vi "Simple TCP - Server - Copy 3 - Copy.vi"() -> ()   [LabVIEW 2021]
doc: "Demonstrates how to set up a basic TCP connection, send data to the specified port once a connection has been established, and terminate the connection once the data has been sent. This VI is designed to stop if the TCP connection is terminated. The data sent in this example is an array of random numbers."
uses:
  <vilib>/Analysis/3filter.llb/Filter Passband Type.ctl
  <vilib>/Analysis/5stat.llb/RMS (DBL).vi
  <vilib>/Analysis/3filter.llb/Butterworth Filter (DBL).vi
  <vilib>/Analysis/NI_AALBase.lvlib
  <vilib>/Analysis/NI_AALPro.lvlib
panel:
  out "Numeric":dbl
  in  "Client Closed":string="The client VI closed the connection."
  out "Waveform Graph":dbl[](graph)
  in  "Stop":bool
  # "Overview: Demonstrates the use of the TCP functions to initialize a TCP server that can send data to a client VI.\nInstructions:\n1. Run the VI.\n2. Open Simple TCP - Client.vi and follow the instructions on its front panel. Note that if you wait longer than 30 seconds to do this after running this VI, it will time out.\n3. Click Stop to stop the VI. Note that if you stop the client VI, this VI will stop automatically."
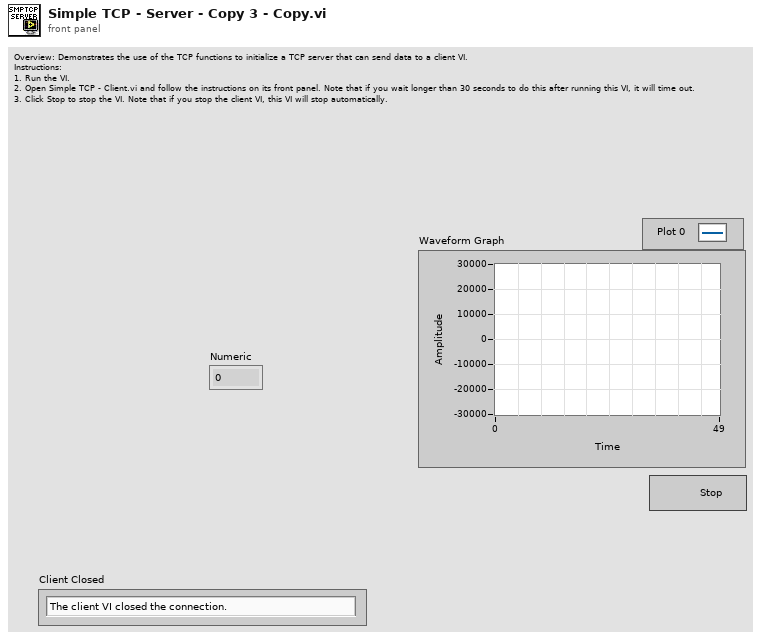
[diagram p1: front panel]
types:
  T1 = typedef "NI_AALBase.lvlib/Filter Passband Type.ctl" = enum32{"Lowpass", "Highpass", "Bandpass", "Bandstop"}
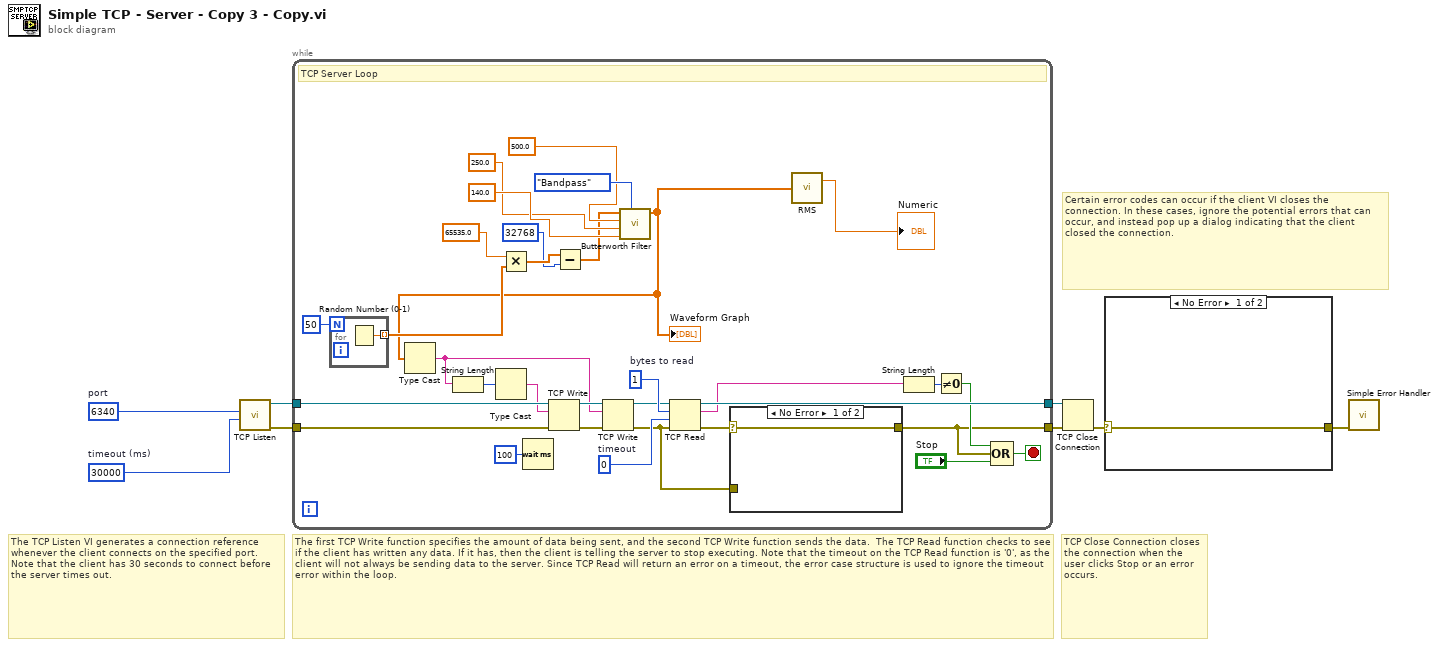
[diagram p0: block diagram]
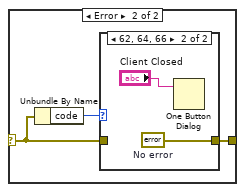
[diagram p2: hidden frame]
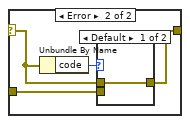
[diagram p4: hidden frame]
diagram:
  w1 = u16 6340  # port
  w2 = 30000  # timeout (ms)
  # "TCP Close Connection closes the connection when the user clicks Stop or an error occurs."
  # "The TCP Listen VI generates a connection reference whenever the client connects on the specified port. Note that the client has 30 seconds to connect before the server times out."
  # "Certain error codes can occur if the client VI closes the connection. In these cases, ignore the potential errors that can occur, and instead pop up a dialog indicating that the client closed the connection."
  # "The first TCP Write function specifies the amount of data being sent, and the second TCP Write function sends the data.  The TCP Read function checks to see if the client has written any data. If it has, then the client is telling the server to stop executing. Note that the timeout on the TCP Read function is '0', as the client will not always be sending data to the server. Since TCP Read will return an error on a timeout, the error case structure is used to ignore the timeout error within the loop."
  n1 = call <vilib>:"TCP Listen.vi"("timeout ms (wait forever: -1)"=w2, "port"=w1) -> ("error out"=w3:errorcluster, "connection ID"=w4:refnum<k5>)  [unwired: 5 in, 3 out]
  n2 = while {
    tunnel: [w21] -> w7
    tunnel: [w27] -> w8
    tunnel: w4 -> [w40]
    tunnel: w3 -> [w31]
    stop <- w33 stop-if-true
    w26 = 0  # timeout
    w29 = 1  # bytes to read
    # "TCP Server Loop"
    n3 = for {
      N: 50 ("# of Points") -> [_]
      tunnel: [w48] -> w12 mode=indexing
      n4 = Random Number (0-1)() -> (number: 0 to 1=w48:dbl)
    }
    n5 = Multiply(x=65535.0 ("x*y"), y=w12) -> (x*y=w19:dbl[])
    n6 = Wait (ms)(milliseconds to wait=u32 100) -> ()  [unwired: 1 out]
    n7 = Subtract(x=w19, y=32768) -> (x-y=w11:dbl[])
    n8 = call-poly <vilib>:"Butterworth Filter.vi"("filter type"=Filter_Passband_Type."Bandpass", "low cutoff freq: fl"=140.0, "high cutoff freq: fh"=250.0, "sampling freq: fs"=500.0, "X"=w11) -> ("Filtered X"=w10:dbl[])  [unwired: 3 in, 1 out]
    "Waveform Graph" <- w10
    n9 = Type Cast(x=w10) -> (*(type *) &x=w35:string)  [unwired: 1 out]
    n10 = String Length(string=w35) -> (length=w37:i32)
    n11 = Type Cast(x=w37) -> (*(type *) &x=w36:string)  [unwired: 1 out]
    n12 = TCP Write(connection ID=w40, data in=w36, error in (no error)=w31) -> (connection ID out=w39:refnum<k5>, error out=w38:errorcluster)  [unwired: 2 out]
    n13 = TCP Write(connection ID=w39, data in=w35, error in (no error)=w38) -> (connection ID out=w28:refnum<k5>, error out=w20:errorcluster)  [unwired: 2 out]
    n14 = TCP Read(connection ID=w28, bytes to read=w29, error in (no error)=w20, 9:w26) -> (connection ID out=w27:refnum<k5>, data out=w24:string, error out=w22:errorcluster)  [unwired: 1 out]
    n15 = case shown="No Error" w22 {
      selector: w22 -> [w41 w44]
      tunnel: [w41 w42] -> w21
      tunnel: w20 -> [_ w43]
      frame No Error {
      }
      frame Error {
        n16 = Unbundle By Name(w44) -> ("code"=w45:i32)
        n17 = case shown="Default" w45 {
          tunnel: w44 -> [w46 _]
          tunnel: w43 -> [_ w47]
          tunnel: [w46 w47] -> w42
          frame Default {
          }
          frame 56 {
          }
        }
      }
    }
    n18 = call-poly <vilib>:"RMS.vi"("X"=w10) -> ("rms value"=→"Numeric":dbl)  [unwired: 1 out]
    n19 = String Length(string=w24) -> (length=w25:i32)
    n20 = Not Equal To 0?(x=w25) -> (x != 0?=w23:bool)
    n21 = Compound Arithmetic op=OR(w23, w21, "Stop") -> (w33:bool)
  }
  n22 = TCP Close Connection(connection ID=w8, error in (no error)=w7) -> (error out=w6:errorcluster)  [unwired: 2 out]
  n23 = case shown="No Error" w6 {
    selector: w6 -> [w49 w51]
    tunnel: [w49 w50] -> w5
    frame No Error {
    }
    frame Error {
      n24 = Unbundle By Name(w51) -> ("code"=w52:i32)
      n25 = case shown="62, 64, 66" w52 {
        tunnel: w51 -> [w53 _]
        tunnel: [w53 w55] -> w50
        frame Default {
        }
        frame 62, 64, 66 {
          w55 = errorcluster {"status"=FALSE, "code"=0, "source"=""}  # No error
          n26 = One Button Dialog(message="Client Closed") -> ()  [unwired: 1 in, 1 out]
        }
      }
    }
  }
  n27 = call <vilib>:"Simple Error Handler.vi"("error in (no error)"=w5) -> ()  [unwired: 1 in, 8 out]
